vi "BRig_dataTrial_T_ENL.vi"() -> (2 "output_T_ENL":i32)   [LabVIEW 2014]
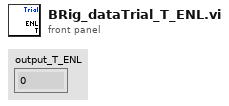
[diagram p1: front panel]
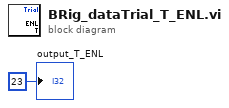
[diagram p0: block diagram]
diagram:
  "output_T_ENL" <- 23 ("output_iBlock")
